vi "DigitalInputs.vi"() -> (0 "NumInputs":u8, 1 "Outputs":u32)   [LabVIEW 2019]
uses:
  <vilib>/rvi/eio/common/nirviEmuTemplateMethod_errors.vi
  <vilib>/eio/EIONode/EIONode.xnode
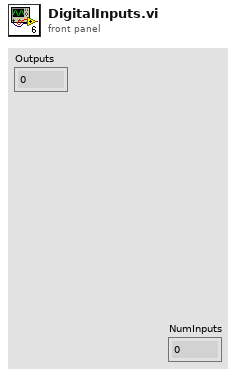
[diagram p1: front panel]
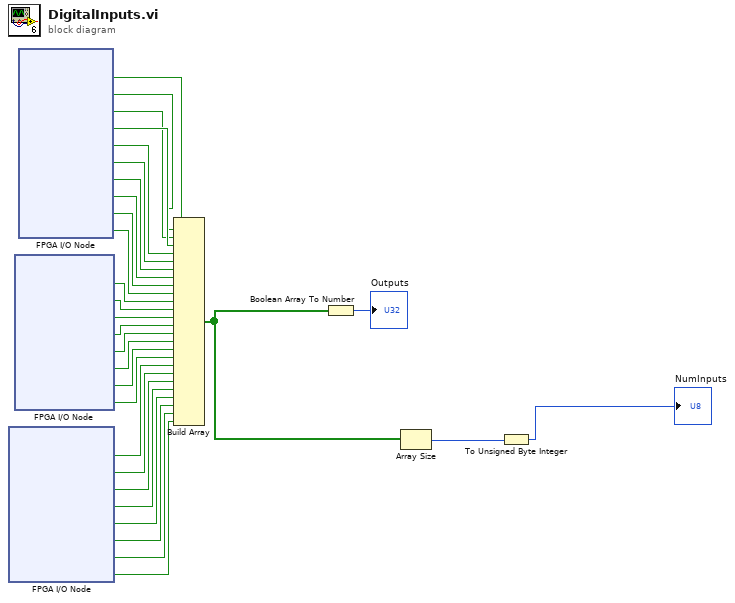
[diagram p0: block diagram]
diagram:
  n1 = xnode "FPGA I/O Node"() -> ("MXP/DIO8"=w16:bool, "MXP/DIO9"=w15:bool, "MXP/DIO10"=w14:bool, "MXP/DIO11"=w13:bool, "MXP/DIO12"=w12:bool, "MXP/DIO13"=w11:bool, "MXP/DIO14"=w10:bool, "MXP/DIO15"=w9:bool)  [unwired: 8 in, 8 out]
  n2 = xnode "FPGA I/O Node"() -> ("MXP/DIO0"=w24:bool, "MXP/DIO1"=w23:bool, "MXP/DIO2"=w22:bool, "MXP/DIO3"=w21:bool, "MXP/DIO4"=w20:bool, "MXP/DIO5"=w19:bool, "MXP/DIO6"=w18:bool, "MXP/DIO7"=w17:bool)  [unwired: 8 in, 8 out]
  n3 = xnode "FPGA I/O Node"() -> ("DIO/DIO0"=w3:bool, "DIO/DIO1"=w4:bool, "DIO/DIO2"=w5:bool, "DIO/DIO3"=w6:bool, "DIO/DIO4"=w30:bool, "DIO/DIO5"=w29:bool, "DIO/DIO6"=w28:bool, "DIO/DIO7"=w27:bool, "DIO/DIO8"=w26:bool, "DIO/DIO9"=w25:bool)  [unwired: 10 in, 10 out]
  n4 = Build Array(w3, w4, w5, w6, w30, w29, w28, w27, w26, w25, w24, w23, w22, w21, w20, w19, w18, w17, w16, w15, w14, w13, w12, w11, w10, w9) -> (w2:bool[])
  n5 = Boolean Array To Number(Boolean array=w2) -> (number=→"Outputs":u32)
  n6 = Array Size(array=w2) -> (size(s)=w8:i32)
  n7 = To Unsigned Byte Integer(number=w8) -> (unsigned 8bit integer=→"NumInputs":u8)
